vi "Anti Defense.vi"(10 "Hue Selector":T2={"Hue"=151.90978129036756, "Saturation"=85.0, "Luminance"=0.0, "Hue Margin"=40.0} {"Hue Margin" scale=0.0..40.0; "Luminance" scale=0.0..255.0; "Saturation" scale=0.0..255.0; "Hue" scale=0.0..255.0}, 11 "New Image":T1) -> (3 "Rectangle":T4)   [LabVIEW 2013]
uses:
  <vilib>/Rock Robotics/WPI/Camera/WPI_CameraFrameRate.ctl
  <vilib>/vision/Image Controls.llb/IMAQ Image.ctl
panel:
  in  "error in (no error)":errorcluster
  in  "Tab Control":enum32{"Simple", "Color Wheel", "HSL Numbers"}(tab)
  in  "Sensitivity":dbl(slide)=2.217391304347826 scale=1.0..5.0
  in  "Basic Color":enum32{"Red", "Green", "Blue"}(radio)=enum."Green"
  in  "AutoCal":bool
  in  "Color Range":T3={"Hue"={"Lower"=55, "Upper"=93}, "Saturation"={"Lower"=73, "Upper"=255}, " Luminance"={"Lower"=99, "Upper"=255}}
  in  "Decimate by":cluster{"H":i32, "V":i32}={"H"=3, "V"=5}
  out "Area":i32
  out "Particles":i32
  out "Mask":T1(plugin-control)
  in  "Frame Rate (fps)":T5=20 min=1 max=30
  # "Determine which color best\ndescribes the target.\n\nMake sure it is in the frame\nand close to the camera,\nthen  press Calibrate.\n\nHigher Sensitivity tightens\nthe fit."
  # "Adjust the color"
  # "You can directly type in HSL threshold numbers.\nThis provides maximum control, but it helps to know\nwhat HSL is. Wikipedia may be able to help with that."
  # "Lower:"
  # "Upper:"
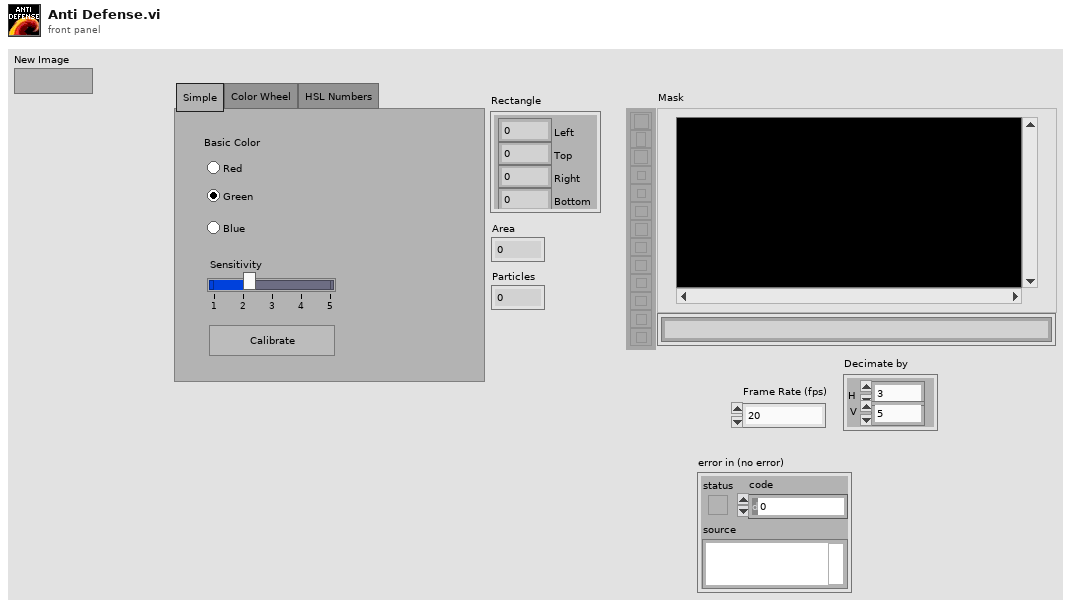
[diagram p1: front panel]
types:
  T1 = typedef "IMAQ Image.ctl" = refnum<image>
  T2 = cluster{"Hue":dbl, "Saturation":dbl, "Luminance":dbl, "Hue Margin":dbl}
  T3 = cluster{"Hue":cluster{"Lower":u8, "Upper":u8}, "Saturation":cluster{"Lower":u8, "Upper":u8}, " Luminance":cluster{"Lower":u8, "Upper":u8}}
  T4 = cluster{"Left":i32, "Top":i32, "Right":i32, "Bottom":i32}
  T5 = typedef "WPI_CameraFrameRate.ctl" = u32
  T6 = cluster{cluster{dbl, dbl}, cluster{"Saturation":dbl, i32}, cluster{"Luminance":dbl, i32}}
  T7 = cluster{cluster{sgl, sgl}, cluster{"Mean Value":sgl, "Standard  Deviation":sgl}}
  T8 = cluster{"Mean Value":sgl, "Standard  Deviation":sgl}
  T9 = cluster{cluster{sgl, sgl}, cluster{sgl, sgl}, cluster{sgl, sgl}}
  T10 = cluster{"Mean Value":sgl, sgl, sgl, "Standard  Deviation":sgl}
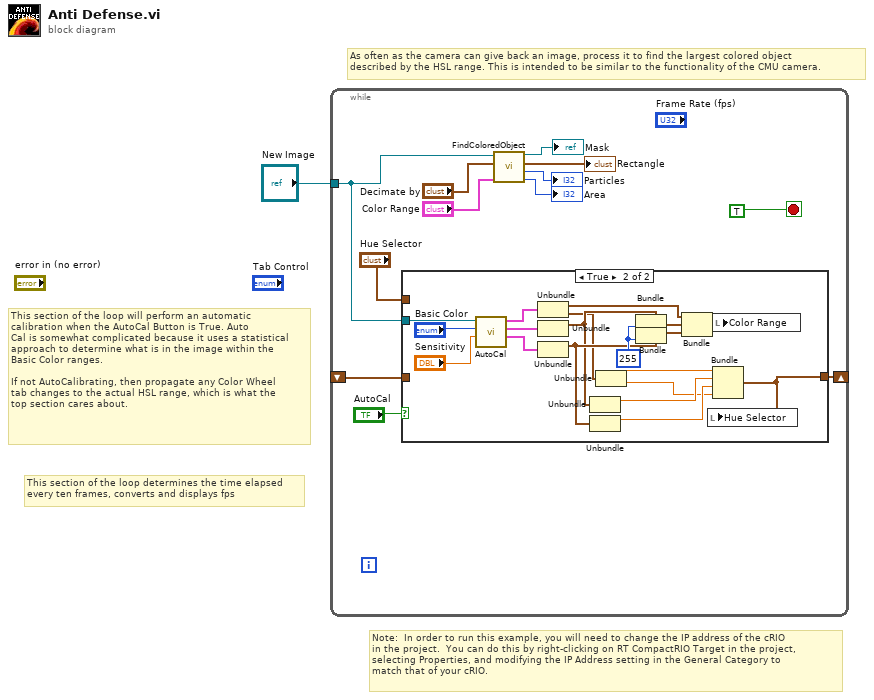
[diagram p0: block diagram]
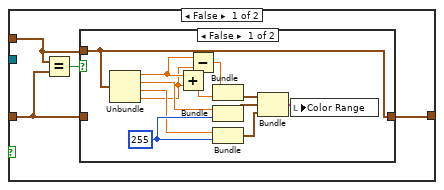
[diagram p2: hidden frame]
diagram:
  # "Note:  In order to run this example, you will need to change the IP address of the cRIO\nin the project.  You can do this by right-clicking on RT CompactRIO Target in the project,\nselecting Properties, and modifying the IP Address setting in the General Category to \nmatch that of your cRIO."
  # "As often as the camera can give back an image, process it to find the largest colored object\ndescribed by the HSL range. This is intended to be similar to the functionality of the CMU camera."
  # "This section of the loop will perform an automatic\ncalibration when the AutoCal Button is True. Auto\nCal is somewhat complicated because it uses a statistical\napproach to determine what is in the image within the\nBasic Color ranges.\n\nIf not AutoCalibrating, then propagate any Color Wheel\ntab changes to the actual HSL range, which is what the\ntop section cares about."
  # "This section of the loop determines the time elapsed\nevery ten frames, converts and displays fps"
  n1 = while {
    tunnel: "New Image" -> [w2]
    shift-right: [w5] -> _
    shift-left: _ -> [w6]
    stop <- TRUE stop-if-true
    n2 = case shown="True" "AutoCal" {
      tunnel: w2 -> [_ w49]
      tunnel: "Hue Selector" -> [w14 _]
      tunnel: w6 -> [w15 _]
      tunnel: [w16 w31] -> w5
      frame False {
        n3 = Equal?(x=w14, y=w15) -> (x = y?=w17:bool)
        n4 = case shown="False" w17 {
          tunnel: w14 -> [w18 _]
          tunnel: [w18 w30] -> w16
          tunnel: w15 -> [_ w30]
          frame False {
            w29 = 255
            n5 = Unbundle(w18) -> ("Hue"=w22:dbl, "Saturation"=w27:dbl, "Luminance"=w28:dbl, "Hue Margin"=w21:dbl)
            n6 = Add(x=w22, y=w21) -> (x+y=w19:dbl)
            n7 = Subtract(x=w22, y=w21) -> (x-y=w20:dbl)
            n8 = Bundle(w20, w19) -> (w24:cluster{dbl, dbl})  [unwired: 1 out]
            n9 = Bundle("Saturation"=w27, w29) -> (w25:cluster{"Saturation":dbl, i32})  [unwired: 1 out]
            n10 = Bundle("Luminance"=w28, w29) -> (w26:cluster{"Luminance":dbl, i32})  [unwired: 1 out]
            n11 = Bundle(w24, w25, w26) -> (w23:T6)  [unwired: 1 out]
            n12 = local write "Color Range"(w23) -> ()
          }
          frame True {
          }
        }
      }
      frame True {
        w39 = 255
        n13 = call "AutoCal.vi"("Std Devs"="Sensitivity", "Target Color"="Basic Color", "Color Image"=w49) -> ("Luminance Info"=w45:T7, "Saturation Info"=w46:T7, "Hue Info"=w48:T7)  [unwired: 6 out]
        n14 = Unbundle(w48) -> (w47:cluster{sgl, sgl}, w34:T8)
        n15 = Unbundle(w46) -> (w36:cluster{sgl, sgl})  [unwired: 1 out]
        n16 = Unbundle(w45) -> (w38:cluster{sgl, sgl})  [unwired: 1 out]
        n17 = Unbundle(w36) -> (w35:sgl)  [unwired: 1 out]
        n18 = Unbundle(w38) -> (w37:sgl)  [unwired: 1 out]
        n19 = Unbundle(w34) -> ("Mean Value"=w32:sgl, "Standard  Deviation"=w33:sgl)
        n20 = Bundle(cluster=w36, w39) -> (w40:cluster{sgl, sgl})  [unwired: 1 out]
        n21 = Bundle(cluster=w38, w39) -> (w41:cluster{sgl, sgl})  [unwired: 1 out]
        n22 = Bundle(w47, w40, w41) -> (w44:T9)  [unwired: 1 out]
        n23 = local write "Color Range"(w44) -> ()
        n24 = Bundle("Mean Value"=w32, w35, w37, "Standard  Deviation"=w33) -> (w31:T10)  [unwired: 1 out]
        n25 = local write "Hue Selector"(w31) -> ()
      }
    }
    n26 = call "FindColoredObject.vi"("Color Range"="Color Range", "Decimate by"="Decimate by", "Color Image In"=w2) -> ("Area"=→"Area":i32, "Particles"=→"Particles":i32, "Rectangle"=→"Rectangle":T4, "Mask Image"=→"Mask":T1)  [unwired: 3 out]
  }
